vi "ExampleSaveFileToMIDASSettingsFileDatabase.vi"() -> ()   [LabVIEW 2018]
uses:
  feGEM DataPacker.lvlib
panel:
  out "MD5 is same":bool
  in  "Send file in this example?":bool
  out "data":string
  out "error out 2":errorcluster
  out "error out":errorcluster
  out "Filename (Local filename is indepentant of the name you want in remote storage)":string
  in  "File":path
  in  "Request Debug Mode":bool
  in  "MIDAS Sever Port":u16=12345
  in  "MIDAS Server":string="my_midas_server.domain"
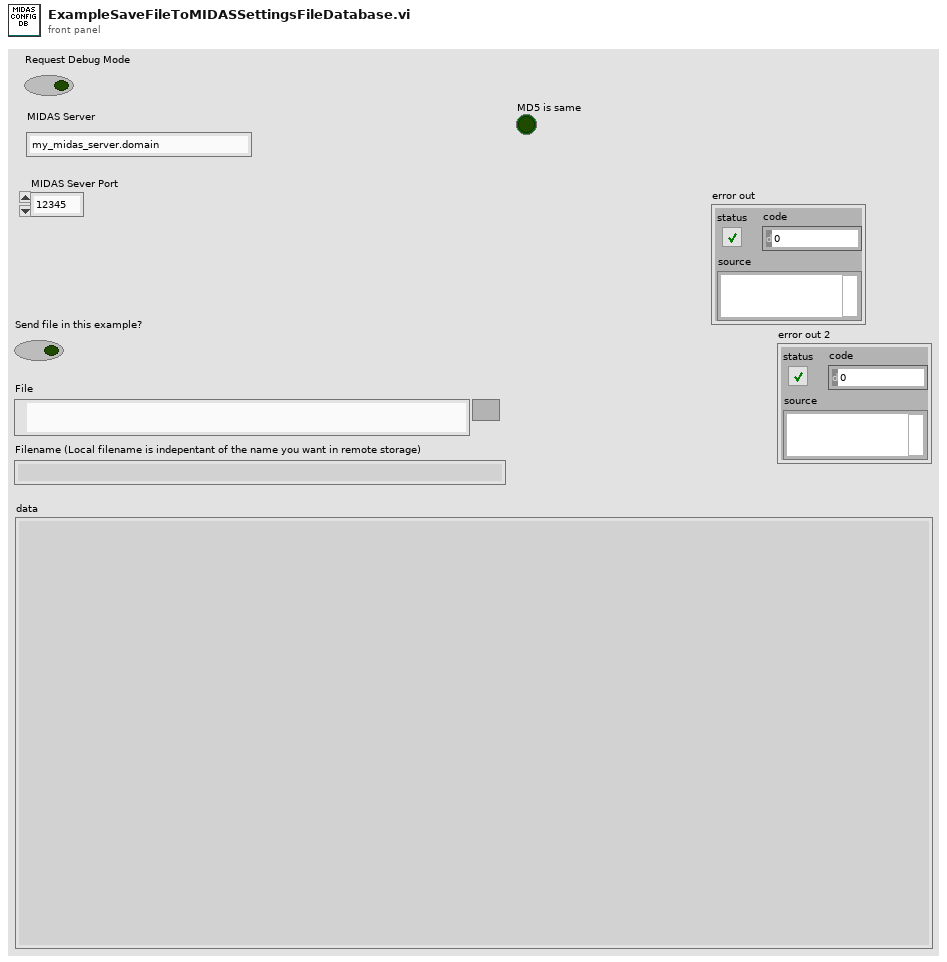
[diagram p1: front panel]
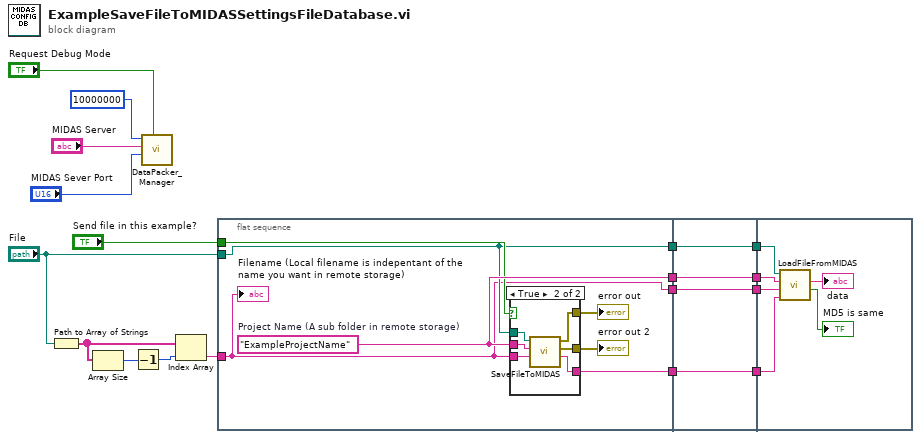
[diagram p0: block diagram]
diagram:
  n1 = Path to Array of Strings(0:"File") -> (2:w6:string[])  [unwired: 1 out]
  n2 = Array Size(array=w6) -> (size(s)=w5:i32)
  n3 = Decrement(x=w5) -> (x-1=w4:i32)
  n4 = call "DataPacker_Manager.vi"("Request Debug Mode"="Request Debug Mode", "MIDAS Sever Port"="MIDAS Sever Port", "MIDAS Server"="MIDAS Server", "Override Max Event size (Data rate bytes/s). Use MIDAS Default = 0"=u32 10000000 ("Override Max Event size (Data rate kb/s). Use MIDAS Default = 0")) -> ()  [unwired: 8 in]
  n5 = Index Array(array=w6, index=w4) -> (element=w3:string)
  n6 = flat-sequence {
    tunnel: [w20] -> w14
    tunnel: [w25] -> w12
    tunnel: [w21] -> w10
    tunnel: "Send file in this example?" -> [w24]
    tunnel: "File" -> [w21]
    tunnel: w3 -> [w20]
    tunnel: [w19] -> w1
    tunnel: w14 -> [w35]
    tunnel: [w35] -> w13
    tunnel: w12 -> [w34]
    tunnel: [w34] -> w11
    tunnel: w10 -> [w33]
    tunnel: [w33] -> w9
    tunnel: [w32] -> w2
    tunnel: w1 -> [w32]
    tunnel: w13 -> [w41]
    tunnel: w11 -> [w40]
    tunnel: w9 -> [w39]
    tunnel: w2 -> [w37]
    frame #0 {
      w25 = "ExampleProjectName"  # Project Name (A sub folder in remote storage)
      n7 = case shown="True" w24 {
        tunnel: [_ w31] -> w23
        tunnel: [_ w30] -> w22
        tunnel: w20 -> [_ w29]
        tunnel: w25 -> [_ w28]
        tunnel: w21 -> [_ w27]
        tunnel: [_ w26] -> w19
        frame False {
        }
        frame True {
          n8 = call "SaveFileToMIDAS.vi"("Filename"=w29, "Project Name"=w28, "File"=w27) -> ("MD5 message-digest"=w26:string, "MD5 Error out"=w30:errorcluster, "Log This Error Out"=w31:errorcluster)  [unwired: 6 in]
        }
      }
      "error out" <- w23
      "error out 2" <- w22
      "Filename (Local filename is indepentant of the name you want in remote storage)" <- w20
    }
    frame #1 {
    }
    frame #2 {
      n9 = call "LoadFileFromMIDAS.vi"("MD5 (optional)"=w37, "Filename"=w41, "Project Name"=w40, "File"=w39) -> ("MD5 is same"=→"MD5 is same":bool, "data"=→"data":string)  [unwired: 6 in]
    }
  }
